vi "Configure1.vi"(8 "error in (no error)":errorcluster, 11 "GRMActor in":refnum<class "DataLoggerUI.lvclass">) -> (0 "error out":errorcluster, 3 "GRMActor out":refnum<class "DataLoggerUI.lvclass">)   [LabVIEW 2020]
uses:
  DataLoggerUI/DataLoggerUI.lvclass
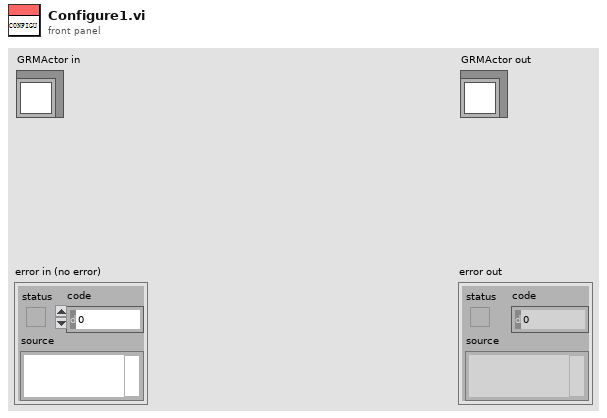
[diagram p1: front panel]
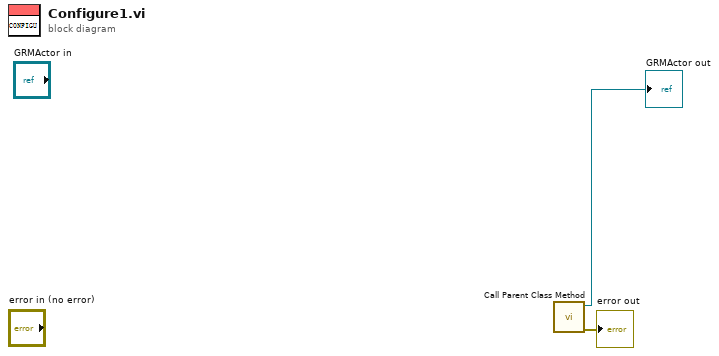
[diagram p0: block diagram]
diagram:
  n1 = call-parent "Call Parent Class Method"() -> ("error out"=→"error out":errorcluster, "GRMActor out"=→"GRMActor out":refnum<class "DataLoggerUI.lvclass">)  [unwired: 10 in]
